vi "PAN_DBS_SetByType.vi"(6 "precision":i8, 7 "queue?":bool, 8 "type":string, 9 "value":string, 10 "name":string, 11 "Database RefNum":T1) -> (1 "response":string)   [LabVIEW 2016]
uses:
  Modules/DBSHAND/private/vis/DatabaseHand_RefNum.ctl
  Modules/DBSHAND/private/vis/DatabaseHand_Element_Set(string).vi
  Modules/DBSHAND/private/vis/DatabaseHand_Element_Set(single).vi
  Modules/DBSHAND/private/vis/DatabaseHand_Element_Set(double).vi
  Modules/DBSHAND/private/vis/DatabaseHand_Element_Set(extended).vi
  Modules/DBSHAND/private/vis/DatabaseHand_Element_Set(I32).vi
  Modules/DBSHAND/private/vis/DatabaseHand_Element_Set(U64).vi
  Modules/DBSHAND/private/vis/DatabaseHand_Element_Set(U32).vi
  Modules/DBSHAND/private/vis/DatabaseHand_Element_Set(I16).vi
  Modules/DBSHAND/private/vis/DatabaseHand_Element_Set(U16).vi
  Modules/DBSHAND/private/vis/DatabaseHand_Element_Set(U8).vi
  Modules/DBSHAND/private/vis/DatabaseHand_Element_Set(I8).vi
  Modules/DBSHAND/private/vis/DatabaseHand_Element_Set(path).vi
  Modules/DBSHAND/private/vis/DatabaseHand_Element_Set(bool).vi
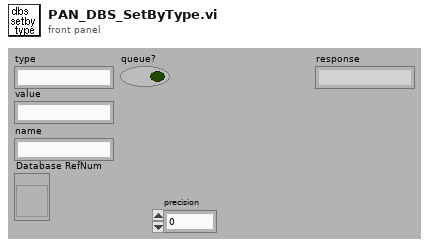
[diagram p1: front panel]
types:
  T1 = typedef "DatabaseHand_RefNum.ctl" = refnum<vi>
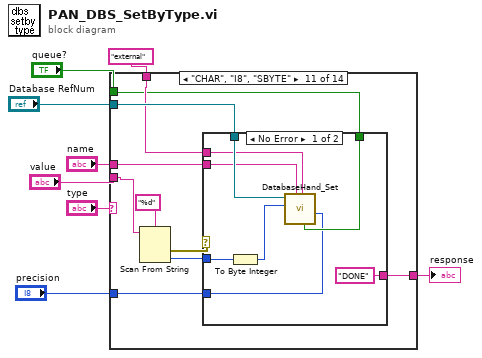
[diagram p0: block diagram]
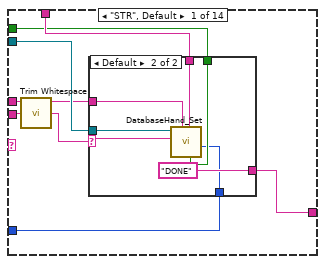
[diagram p2: hidden frame]
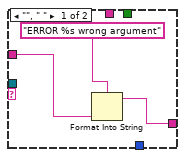
[diagram p3: hidden frame]
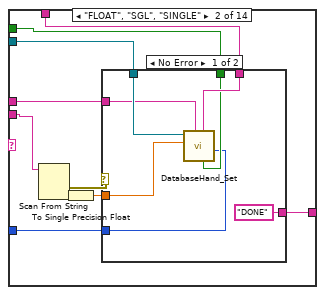
[diagram p4: hidden frame]
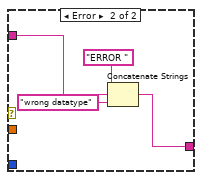
[diagram p5: hidden frame]
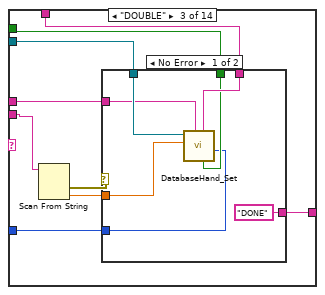
[diagram p6: hidden frame]
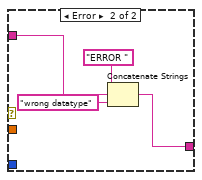
[diagram p7: hidden frame]
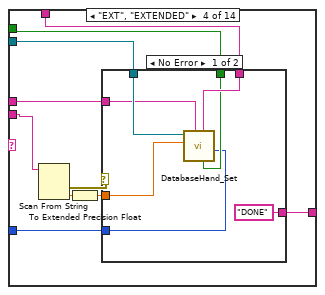
[diagram p8: hidden frame]
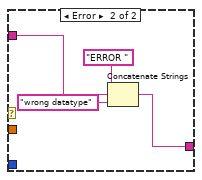
[diagram p9: hidden frame]
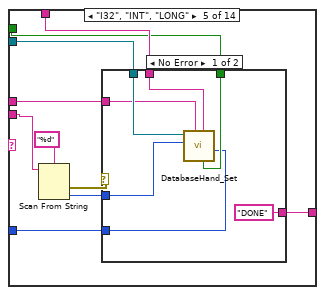
[diagram p10: hidden frame]
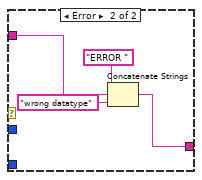
[diagram p11: hidden frame]
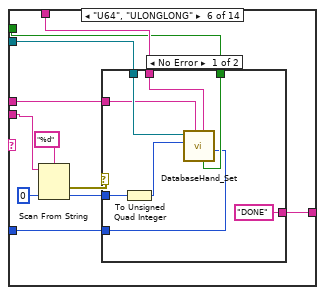
[diagram p12: hidden frame]
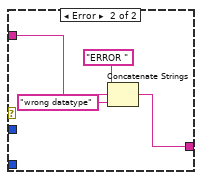
[diagram p13: hidden frame]
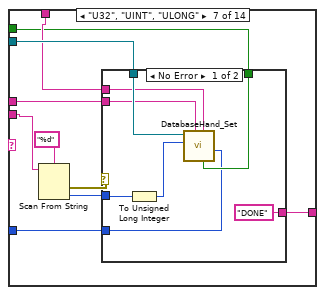
[diagram p14: hidden frame]
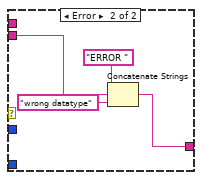
[diagram p15: hidden frame]
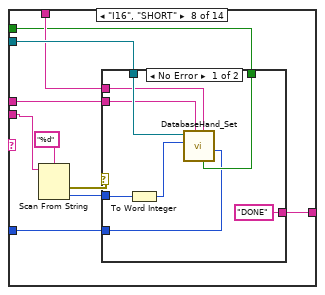
[diagram p16: hidden frame]
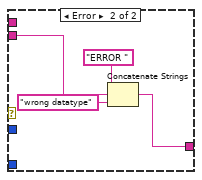
[diagram p17: hidden frame]
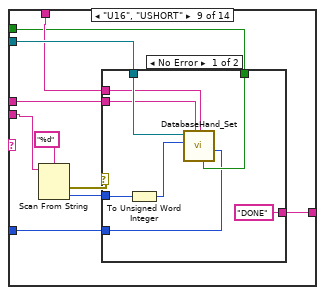
[diagram p18: hidden frame]
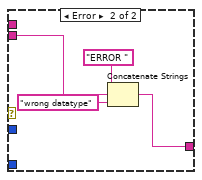
[diagram p19: hidden frame]
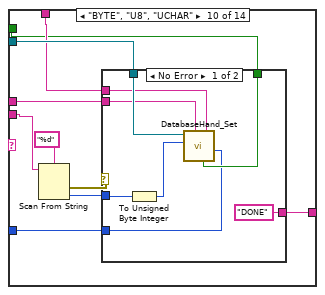
[diagram p20: hidden frame]
diagram:
  n1 = case shown="\"CHAR\", \"I8\", \"SBYTE\"" "type" {
    tunnel: "Database RefNum" -> [w16 w32 w53 w74 w94 w116 w138 w160 w182 w204 w226 w248 w270 _]
    tunnel: "value" -> [w15 w34 w55 w76 w96 w118 w140 w162 w184 w206 w228 w250 w272 _]
    tunnel: "name" -> [w14 w31 w52 w73 w93 w115 w137 w159 w181 w203 w225 w247 w269 _]
    tunnel: [w11 w33 w54 w75 w95 w117 w139 w161 w183 w205 w227 w249 w271 "ERROR unknown variable, must provide type at the end " ("source")] -> w2
    tunnel: "external" ("group") -> [w13 w30 w51 w72 w91 w113 w135 w157 w179 w201 w223 w245 w267 _]
    tunnel: "queue?" -> [w10 w28 w49 w70 w90 w112 w134 w156 w178 w200 w222 w244 w266 _]
    tunnel: "precision" -> [w9 w27 w48 w68 w89 w110 w133 w155 w177 w199 w221 w243 w265 _]
    frame "STR", Default {
      n2 = call <vilib>:"Trim Whitespace.vi"("string"=w15) -> ("trimmed string"=w12:string)  [unwired: 1 in]
      n3 = case shown="Default" w12 {
        selector: w12 -> [_ w23]
        tunnel: w16 -> [_ w26]
        tunnel: w14 -> [w18 w25]
        tunnel: w13 -> [_ w24]
        tunnel: [w17 "DONE" ("source")] -> w11
        tunnel: w10 -> [_ w21]
        tunnel: w9 -> [_ w20]
        frame "", " " {
          n4 = Format Into String(format string="ERROR %s wrong argument", w18) -> (resulting string=w17:string)  [unwired: 2 in, 1 out]
        }
        frame Default {
          n5 = call-poly "DatabaseHand_Set.vi"("precision"=w20, "enqueue? (F)"=w21, "group"=w24, "name"=w25, "value"=w23, "Database RefNum in"=w26) -> ()  [unwired: 3 in, 3 out]
        }
      }
    }
    frame "FLOAT", "SGL", "SINGLE" {
      n6 = Scan From String(input string=w34) -> (error out=w36:errorcluster, output 1=w35:dbl)  [unwired: 3 in, 3 out]
      n7 = To Single Precision Float(number=w35) -> (single precision float=w29:sgl)
      n8 = case shown="No Error" w36 {
        tunnel: w29 -> [w41 _]
        tunnel: ["DONE" w44] -> w33
        tunnel: w32 -> [w42 _]
        tunnel: w31 -> [w40 w46]
        tunnel: w30 -> [w39 _]
        tunnel: w28 -> [w38 _]
        tunnel: w27 -> [w37 _]
        frame No Error {
          n9 = call-poly "DatabaseHand_Set.vi"("precision"=w37, "enqueue? (F)"=w38, "group"=w39, "name"=w40, "value"=w41, "Database RefNum in"=w42) -> ()  [unwired: 3 in, 3 out]
        }
        frame Error {
          n10 = Concatenate Strings("ERROR " ("string"), w46, "wrong datatype" ("string")) -> (w44:string)
        }
      }
    }
    frame "DOUBLE" {
      n11 = Scan From String(input string=w55) -> (error out=w56:errorcluster, output 1=w50:dbl)  [unwired: 3 in, 3 out]
      n12 = case shown="No Error" w56 {
        tunnel: w50 -> [w61 _]
        tunnel: ["DONE" w64] -> w54
        tunnel: w53 -> [w62 _]
        tunnel: w52 -> [w60 w66]
        tunnel: w51 -> [w59 _]
        tunnel: w49 -> [w58 _]
        tunnel: w48 -> [w57 _]
        frame No Error {
          n13 = call-poly "DatabaseHand_Set.vi"("precision"=w57, "enqueue? (F)"=w58, "group"=w59, "name"=w60, "value"=w61, "Database RefNum in"=w62) -> ()  [unwired: 3 in, 3 out]
        }
        frame Error {
          n14 = Concatenate Strings("ERROR " ("string"), w66, "wrong datatype" ("string")) -> (w64:string)
        }
      }
    }
    frame "EXT", "EXTENDED" {
      n15 = Scan From String(input string=w76) -> (error out=w77:errorcluster, output 1=w71:dbl)  [unwired: 3 in, 3 out]
      n16 = To Extended Precision Float(1:w71) -> (0:w69:ext)
      n17 = case shown="No Error" w77 {
        tunnel: w69 -> [w82 _]
        tunnel: ["DONE" w85] -> w75
        tunnel: w74 -> [w83 _]
        tunnel: w73 -> [w81 w87]
        tunnel: w72 -> [w80 _]
        tunnel: w70 -> [w79 _]
        tunnel: w68 -> [w78 _]
        frame No Error {
          n18 = call-poly "DatabaseHand_Set.vi"("precision"=w78, "enqueue? (F)"=w79, "group"=w80, "name"=w81, "value"=w82, "Database RefNum in"=w83) -> ()  [unwired: 3 in, 3 out]
        }
        frame Error {
          n19 = Concatenate Strings("ERROR " ("string"), w87, "wrong datatype" ("string")) -> (w85:string)
        }
      }
    }
    frame "I32", "INT", "LONG" {
      n20 = Scan From String(format string="%d", input string=w96) -> (error out=w98:errorcluster, output 1=w97:i32)  [unwired: 2 in, 3 out]
      n21 = case shown="No Error" w98 {
        tunnel: w97 -> [w103 _]
        tunnel: ["DONE" w106] -> w95
        tunnel: w94 -> [w104 _]
        tunnel: w93 -> [w102 w108]
        tunnel: w91 -> [w101 _]
        tunnel: w90 -> [w100 _]
        tunnel: w89 -> [w99 _]
        frame No Error {
          n22 = call-poly "DatabaseHand_Set.vi"("precision"=w99, "enqueue? (F)"=w100, "group"=w101, "name"=w102, "value"=w103, "Database RefNum in"=w104) -> ()  [unwired: 3 in, 3 out]
        }
        frame Error {
          n23 = Concatenate Strings("ERROR " ("string"), w108, "wrong datatype" ("string")) -> (w106:string)
        }
      }
    }
    frame "U64", "ULONGLONG" {
      n24 = Scan From String(format string="%d", input string=w118, default 1=u64 0 ("default value 1")) -> (error out=w120:errorcluster, output 1=w119:u64)  [unwired: 2 in, 2 out]
      n25 = case shown="No Error" w120 {
        tunnel: w119 -> [w126 _]
        tunnel: ["DONE" w129] -> w117
        tunnel: w116 -> [w127 _]
        tunnel: w115 -> [w125 w131]
        tunnel: w113 -> [w124 _]
        tunnel: w112 -> [w123 _]
        tunnel: w110 -> [w121 _]
        frame No Error {
          n26 = To Unsigned Quad Integer(1:w126) -> (0:w122:u64)
          n27 = call-poly "DatabaseHand_Set.vi"("precision"=w121, "enqueue? (F)"=w123, "group"=w124, "name"=w125, "value"=w122, "Database RefNum in"=w127) -> ()  [unwired: 3 in, 3 out]
        }
        frame Error {
          n28 = Concatenate Strings("ERROR " ("string"), w131, "wrong datatype" ("string")) -> (w129:string)
        }
      }
    }
    frame "U32", "UINT", "ULONG" {
      n29 = Scan From String(format string="%d", input string=w140) -> (error out=w142:errorcluster, output 1=w141:i32)  [unwired: 2 in, 3 out]
      n30 = case shown="No Error" w142 {
        tunnel: w141 -> [w147 _]
        tunnel: ["DONE" w151] -> w139
        tunnel: w138 -> [w149 _]
        tunnel: w137 -> [w146 w153]
        tunnel: w135 -> [w145 _]
        tunnel: w134 -> [w144 _]
        tunnel: w133 -> [w143 _]
        frame No Error {
          n31 = To Unsigned Long Integer(number=w147) -> (unsigned 32bit integer=w148:u32)
          n32 = call-poly "DatabaseHand_Set.vi"("precision"=w143, "enqueue? (F)"=w144, "group"=w145, "name"=w146, "value"=w148, "Database RefNum in"=w149) -> ()  [unwired: 3 in, 3 out]
        }
        frame Error {
          n33 = Concatenate Strings("ERROR " ("string"), w153, "wrong datatype" ("string")) -> (w151:string)
        }
      }
    }
    frame "I16", "SHORT" {
      n34 = Scan From String(format string="%d", input string=w162) -> (error out=w164:errorcluster, output 1=w163:i32)  [unwired: 2 in, 3 out]
      n35 = case shown="No Error" w164 {
        tunnel: w163 -> [w169 _]
        tunnel: ["DONE" w173] -> w161
        tunnel: w160 -> [w171 _]
        tunnel: w159 -> [w168 w175]
        tunnel: w157 -> [w167 _]
        tunnel: w156 -> [w166 _]
        tunnel: w155 -> [w165 _]
        frame No Error {
          n36 = To Word Integer(number=w169) -> (16bit integer=w170:i16)
          n37 = call-poly "DatabaseHand_Set.vi"("precision"=w165, "enqueue? (F)"=w166, "group"=w167, "name"=w168, "value"=w170, "Database RefNum in"=w171) -> ()  [unwired: 3 in, 3 out]
        }
        frame Error {
          n38 = Concatenate Strings("ERROR " ("string"), w175, "wrong datatype" ("string")) -> (w173:string)
        }
      }
    }
    frame "U16", "USHORT" {
      n39 = Scan From String(format string="%d", input string=w184) -> (error out=w186:errorcluster, output 1=w185:i32)  [unwired: 2 in, 3 out]
      n40 = case shown="No Error" w186 {
        tunnel: w185 -> [w191 _]
        tunnel: ["DONE" w195] -> w183
        tunnel: w182 -> [w193 _]
        tunnel: w181 -> [w190 w197]
        tunnel: w179 -> [w189 _]
        tunnel: w178 -> [w188 _]
        tunnel: w177 -> [w187 _]
        frame No Error {
          n41 = To Unsigned Word Integer(number=w191) -> (unsigned 16bit integer=w192:u16)
          n42 = call-poly "DatabaseHand_Set.vi"("precision"=w187, "enqueue? (F)"=w188, "group"=w189, "name"=w190, "value"=w192, "Database RefNum in"=w193) -> ()  [unwired: 3 in, 3 out]
        }
        frame Error {
          n43 = Concatenate Strings("ERROR " ("string"), w197, "wrong datatype" ("string")) -> (w195:string)
        }
      }
    }
    frame "BYTE", "U8", "UCHAR" {
      n44 = Scan From String(format string="%d", input string=w206) -> (error out=w208:errorcluster, output 1=w207:i32)  [unwired: 2 in, 3 out]
      n45 = case shown="No Error" w208 {
        tunnel: w207 -> [w213 _]
        tunnel: ["DONE" w217] -> w205
        tunnel: w204 -> [w215 _]
        tunnel: w203 -> [w212 w219]
        tunnel: w201 -> [w211 _]
        tunnel: w200 -> [w210 _]
        tunnel: w199 -> [w209 _]
        frame No Error {
          n46 = To Unsigned Byte Integer(number=w213) -> (unsigned 8bit integer=w214:u8)
          n47 = call-poly "DatabaseHand_Set.vi"("precision"=w209, "enqueue? (F)"=w210, "group"=w211, "name"=w212, "value"=w214, "Database RefNum in"=w215) -> ()  [unwired: 3 in, 3 out]
        }
        frame Error {
          n48 = Concatenate Strings("ERROR " ("string"), w219, "wrong datatype" ("string")) -> (w217:string)
        }
      }
    }
    frame "CHAR", "I8", "SBYTE" {
      n49 = Scan From String(format string="%d", input string=w228) -> (error out=w230:errorcluster, output 1=w229:i32)  [unwired: 2 in, 3 out]
      n50 = case shown="No Error" w230 {
        tunnel: w229 -> [w235 _]
        tunnel: ["DONE" w239] -> w227
        tunnel: w226 -> [w237 _]
        tunnel: w225 -> [w234 w241]
        tunnel: w223 -> [w233 _]
        tunnel: w222 -> [w232 _]
        tunnel: w221 -> [w231 _]
        frame No Error {
          n51 = To Byte Integer(number=w235) -> (8bit integer=w236:i8)
          n52 = call-poly "DatabaseHand_Set.vi"("precision"=w231, "enqueue? (F)"=w232, "group"=w233, "name"=w234, "value"=w236, "Database RefNum in"=w237) -> ()  [unwired: 3 in, 3 out]
        }
        frame Error {
          n53 = Concatenate Strings("ERROR " ("string"), w241, "wrong datatype" ("string")) -> (w239:string)
        }
      }
    }
    frame "PATH" {
      n54 = Scan From String(format string="%s", input string=w250) -> (error out=w252:errorcluster, output 1=w251:string)  [unwired: 2 in, 3 out]
      n55 = case shown="No Error" w252 {
        tunnel: w251 -> [w256 _]
        tunnel: ["DONE" w261] -> w249
        tunnel: w248 -> [w259 _]
        tunnel: w247 -> [w258 w263]
        tunnel: w245 -> [w257 _]
        tunnel: w244 -> [w254 _]
        tunnel: w243 -> [w253 _]
        frame No Error {
          n56 = String To Path(string=w256) -> (path=w255:path)
          n57 = call-poly "DatabaseHand_Set.vi"("precision"=w253, "enqueue? (F)"=w254, "group"=w257, "name"=w258, "value"=w255, "Database RefNum in"=w259) -> ()  [unwired: 3 in, 3 out]
        }
        frame Error {
          n58 = Concatenate Strings("ERROR " ("string"), w263, "wrong argument" ("string")) -> (w261:string)
        }
      }
    }
    frame "BIT", "BOOL" {
      n59 = Scan From String(format string="%s", input string=w272) -> (error out=w274:errorcluster, output 1=w273:string)  [unwired: 2 in, 3 out]
      n60 = case shown="No Error" w274 {
        tunnel: w273 -> [w280 _]
        tunnel: [w277 w298] -> w271
        tunnel: w270 -> [w281 _]
        tunnel: w269 -> [w278 w300]
        tunnel: w267 -> [w279 _]
        tunnel: w266 -> [w276 _]
        tunnel: w265 -> [w275 _]
        frame No Error {
          n61 = case shown="\"on\", \"true\", \"yes\"" w280 {
            tunnel: w281 -> [_ w291 w297]
            tunnel: w279 -> [_ w290 w296]
            tunnel: w278 -> [w283 w289 w295]
            tunnel: [w282 "DONE" "DONE"] -> w277
            tunnel: w276 -> [_ w286 w292]
            tunnel: w275 -> [_ w285 _]
            frame Default {
              n62 = Format Into String(format string="ERROR %s wrong argument", w283) -> (resulting string=w282:string)  [unwired: 2 in, 1 out]
            }
            frame "on", "true", "yes" {
              n63 = call-poly "DatabaseHand_Set.vi"("precision"=w285, "enqueue? (F)"=w286, "group"=w290, "name"=w289, "value"=TRUE, "Database RefNum in"=w291) -> ()  [unwired: 3 in, 3 out]
            }
            frame "false", "no", "off" {
              n64 = call-poly "DatabaseHand_Set.vi"("enqueue? (F)"=w292, "group"=w296, "name"=w295, "value"=FALSE, "Database RefNum in"=w297) -> ()  [unwired: 3 in, 4 out]
            }
          }
        }
        frame Error {
          n65 = Concatenate Strings("ERROR " ("string"), w300, "wrong datatype" ("string")) -> (w298:string)
        }
      }
    }
    frame "", " " {
    }
  }
  "response" <- w2
